vi "Inst.RP100.Public API.vi"(8 "error in (no error)":errorcluster, 11 "Inst.RP100 in":refnum<class "Inst.RP100.lvclass">) -> (0 "error out":errorcluster, 2 "commands (this level)":string[](array[string]), 3 "Inst.RP100 out":refnum<class "Inst.RP100.lvclass">)   [LabVIEW 2019, in "Inst.RP100.lvlib" / "Inst.RP100.lvclass"]
doc: "Override this VI to return a list of commands only supported by your Instrument"
uses:
  Inst.RP100.lvclass
  Typedefs/Inst.RP100.Commands--Enum.ctl
  a4aa464b-495f-48b8-8854-29107d0a4bf0.vi
  <vilib>/Utility/Data Type/Get Type Information.vi
  <vilib>/Utility/Data Type/Get Numeric Information.vi
  <userlib>/_OpenG.lib/lvdata/lvdata.llb/Unwrap VVariant__ogtk.vi
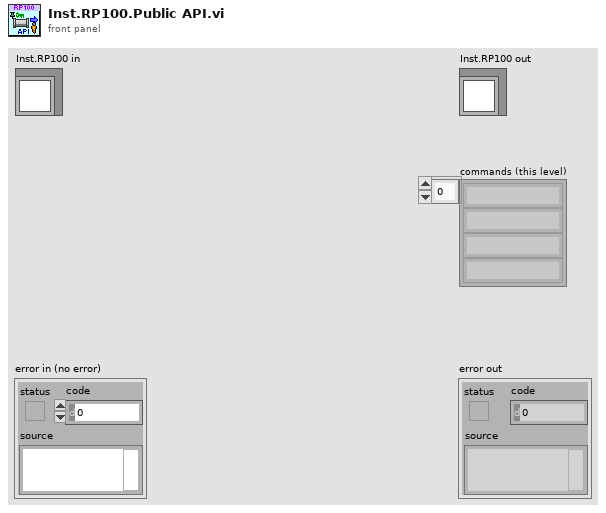
[diagram p1: front panel]
types:
  T1 = typedef "Inst.RP100.lvlib/Inst.RP100.lvclass/Inst.RP100.Commands--Enum.ctl" = enum16{"setState", "setLevel", "getLevel"}
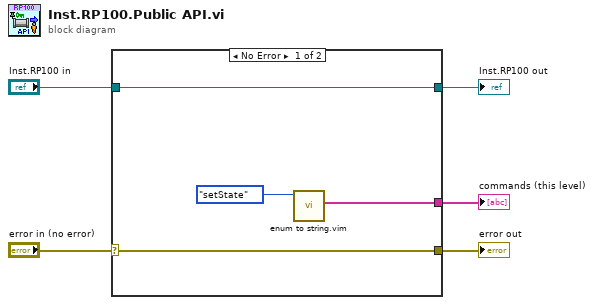
[diagram p0: block diagram]
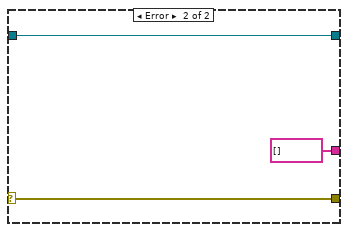
[diagram p2: hidden frame]
diagram:
  n1 = case shown="No Error" "error in (no error)" {
    selector: "error in (no error)" -> [w8 w12]
    tunnel: [w6 string[] []] -> w5
    tunnel: [w8 w12] -> w4
    tunnel: [w7 w10] -> w2
    tunnel: "Inst.RP100 in" -> [w7 w10]
    frame No Error {
      n2 = call "enum to string.vim"("enum in"=Inst.RP100.Commands--Enum."setState" ("Commands")) -> ("strings out"=w6:string[])  [unwired: 9 in, 1 out]
    }
    frame Error {
    }
  }
  "error out" <- w4
  "Inst.RP100 out" <- w2
  "commands (this level)" <- w5
